vi "RCServo TargetPositionReachedEvent Example.vi"() -> ()   [LabVIEW 2012, in "Phidget RC Servo.lvlib"]
uses:
  <instrlib>/Phidgets/Phidget RC Servo/Phidget RC Servo.lvlib
  <instrlib>/Phidgets/Phidget RC Servo/Public/RCServoStart.vi
  <instrlib>/Phidgets/Phidget RC Servo/Public/RCServoClose.vi
  <instrlib>/Phidgets/Phidget Common/Phidget Common.lvlib
panel:
  in  "RCServo Initialization Data":T1={"Velocity Limit"=180.0, "Acceleration"=360.0, "Min PW"=550, "Max PW"=2350, "Max Position"=180.0, "Min Position"=0.0, "Speed Ramping State"=TRUE}
  out "Position":dbl format="%.2f"
  in  "stop":bool
  out "Serial Number Return":i32
  in  "Device Info":T2={"Serial Number"=-1, "Channel"=0, "Port"=0}
  out "error out":errorcluster
  # "Be sure to use this stop button to stop the program.\nIf you use the \"Abort Execution\" button, you will\nneed to use PhidgetResetLibrary.vi or restart Labview \nin order for any Phidgets to work."
  # "Enabled\n\nDisabled"
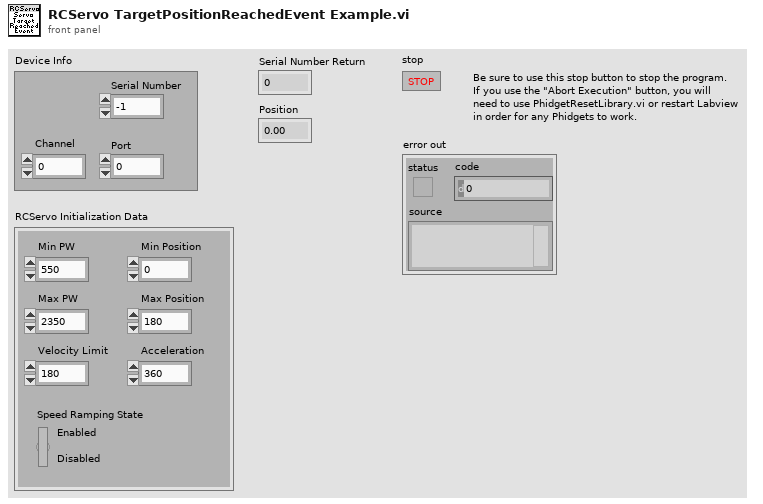
[diagram p1: front panel]
types:
  T1 = cluster{"Velocity Limit":dbl, "Acceleration":dbl, "Min PW":i32, "Max PW":i32, "Max Position":dbl, "Min Position":dbl, "Speed Ramping State":bool}
  T2 = cluster{"Serial Number":i32, "Channel":i32, "Port":i32}
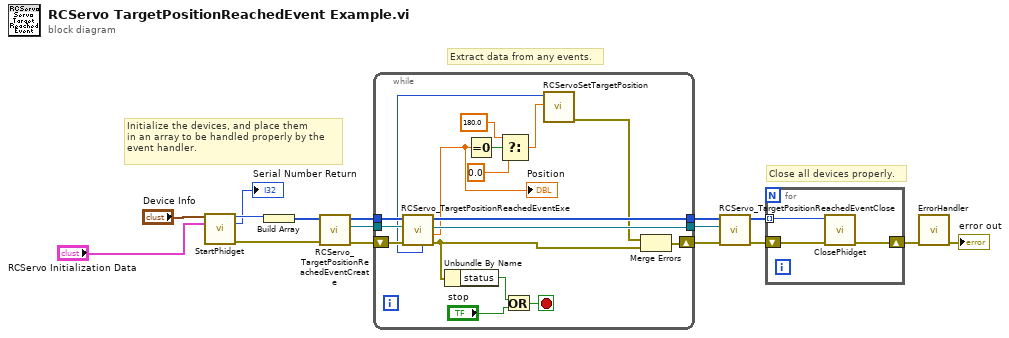
[diagram p0: block diagram]
diagram:
  # "Close all devices properly."
  # "Extract data from any events."
  # "Initialize the devices, and place them\nin an array to be handled properly by the\nevent handler."
  n1 = call-poly <instrlib>:"StartPhidget.vi"("Device Info"="Device Info", "RCServo Initialization Data"="RCServo Initialization Data") -> ("Phidget ID"=w4:u64, "Serial Number Return"=→"Serial Number Return":i32, "error out"=w2:errorcluster)  [unwired: 10 in, 1 out]
  n2 = Build Array(w4) -> (w16:u64[])
  n3 = call <instrlib>:"RCServo_TargetPositionReachedEventCreate.vi"("error in (no error)"=w2, "Devices In"=w16) -> ("error out"=w9:errorcluster, "Event Registration Refnum"=w14:refnum<event-registration>, "Devices Out"=w15:u64[])  [unwired: 7 in]
  n4 = while {
    tunnel: w15 -> [w33]
    tunnel: w14 -> [w29]
    tunnel: [w32] -> w11
    shift-right: [w24] -> w10
    shift-left: w9 -> [w31]
    tunnel: [w30] -> w5
    stop <- w28 stop-if-true
    n5 = call <instrlib>:"RCServo_TargetPositionReachedEventExe.vi"("error in (no error)"=w31, "Event Registration Refnum In"=w29, "Devices In"=w33) -> ("error out"=w25:errorcluster, "Position"=w18:dbl, "Event Registration Refnum Out"=w32:refnum<event-registration>, "Devices Out"=w30:u64[], "phid"=w19:u64)  [unwired: 2 in, 2 out]
    "Position" <- w18
    n6 = Unbundle By Name(w25) -> ("status"=w26:bool)
    n7 = Equal To 0?(x=w18) -> (x = 0?=w23:bool)
    n8 = Select(t=180.0, s=w23, f=0.0) -> (s? t:f=w20:dbl)
    n9 = Or(x=w26, y="stop") -> (x .or. y?=w28:bool)
    n10 = call <instrlib>:"RCServoSetTargetPosition.vi"("Target Position"=w20, "Device In"=w19) -> ("error out"=w17:errorcluster)  [unwired: 7 in, 1 out]
    n11 = Merge Errors(w17, w25) -> (w24:errorcluster)
  }
  n12 = call <instrlib>:"RCServo_TargetPositionReachedEventClose.vi"("error in (no error)"=w10, "Event Registration Refnum In"=w11, "Devices In"=w5) -> ("error out"=w7:errorcluster, "Devices Out"=w6:u64[])  [unwired: 7 in]
  n13 = for {
    tunnel: w6 -> [w34] mode=indexing
    shift-right: [w36] -> w13
    shift-left: w7 -> [w35]
    n14 = call-poly <instrlib>:"ClosePhidget.vi"("error in"=w35, "Device In"=w34) -> ("error out"=w36:errorcluster)  [unwired: 9 in]
  }
  n15 = call <instrlib>:"ErrorHandler.vi"("error in"=w13) -> ("error out"=→"error out":errorcluster)  [unwired: 9 in, 1 out]
